vi "MGC_Device.vi"(8 "Error in":errorcluster, 9 "Port":i32=7, 10 "IPAddress":string) -> (0 "Error out":errorcluster, 3 "Device":refnum<k24>)   [LabVIEW 2016]
doc: "Generates a new MGC device.\n\nIPAddress: IPAddress of the device you want to connect with\nPort: Port of the device you want to connect with (default port is 7)"
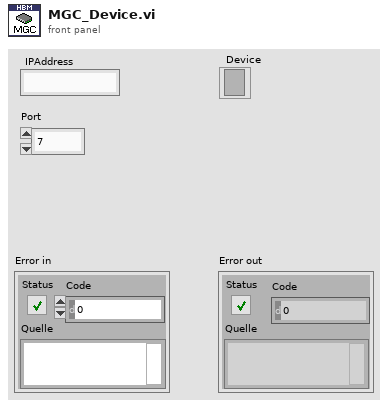
[diagram p1: front panel]
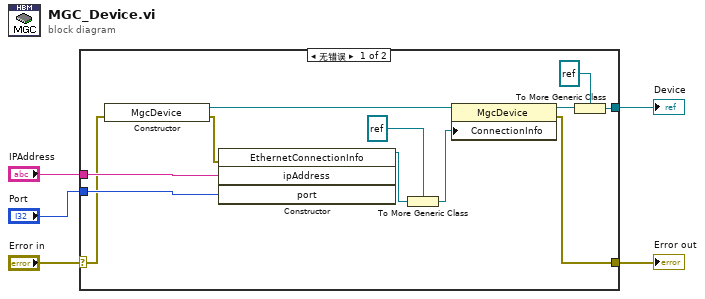
[diagram p0: block diagram]
diagram:
  n1 = case shown="无错误" "Error in" {
    selector: "Error in" -> [w11 w18]
    tunnel: "IPAddress" -> [w17 _]
    tunnel: "Port" -> [w16 _]
    tunnel: [w10 w18] -> w2
    tunnel: [w12 _] -> w1
    frame No Error {
      n2 = constructor class="MgcDevice"(error in=w11) -> (reference out=w14:refnum<k24>, error out=w15:errorcluster)  [unwired: 2 in, 1 out]
      n3 = constructor class="EthernetConnectionInfo"(error in=w15, "ipAddress"=w17, "port"=w16) -> (reference out=w8:refnum<k24>)  [unwired: 2 in, 4 out]
      n4 = To More Generic Class(target class=refnum<k24> refnum (".NET (Referenz)"), reference=w8) -> (generic class reference=w7:refnum<k24>)
      n5 = property on="Eigenschaftsknoten" class="MgcDevice"(reference=w14, "ConnectionInfo"=w7) -> (reference out=w13:refnum<k24>, error out=w10:errorcluster)  [unwired: 1 in]
      n6 = To More Generic Class(target class=refnum<k24> refnum (".NET (Referenz)"), reference=w13) -> (generic class reference=w12:refnum<k24>)
    }
    frame Error {
    }
  }
  "Error out" <- w2
  "Device" <- w1
